vi "WaveFormDataGenerator.vi"(8 "error in":errorcluster, 9 "sampling info":cluster{"Fs":dbl, "#s":dbl}={"Fs"=1000.0, "#s"=100.0}, 10 "Signal Types/Classes":T1(array[ring])=[enum."Sine Wave", enum."Square Wave", enum."Triangle Wave"], 11 "Number of Waveforms per Signal Type":i32=2500) -> (0 "error out":errorcluster, 2 "One-Hot Encoded Labels":sgl[][](array[numeric]), 3 "Generated Waveform":sgl[][](array[numeric]))   [LabVIEW 2020]
uses:
  <vilib>/numeric/Random Number (Range) DBL.vi
  <vilib>/measure/NI_MABase.lvlib
  <vilib>/Ngene/DeepLTK/Toolkit/Deep_Learning_Toolkit_by_Ngene.lvlib
panel:
  out "Class Indices":i32[](array[numeric])
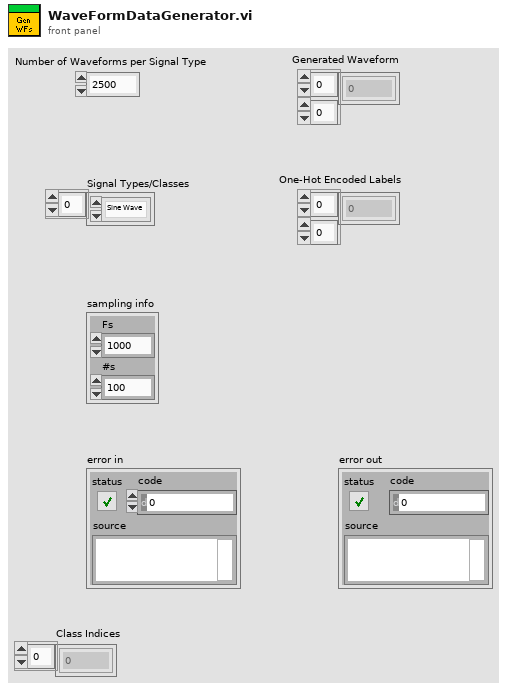
[diagram p1: front panel]
types:
  T1 = enum16{"Sine Wave", "Triangle Wave", "Square Wave", "Sawtooth Wave", "Noise"}[]
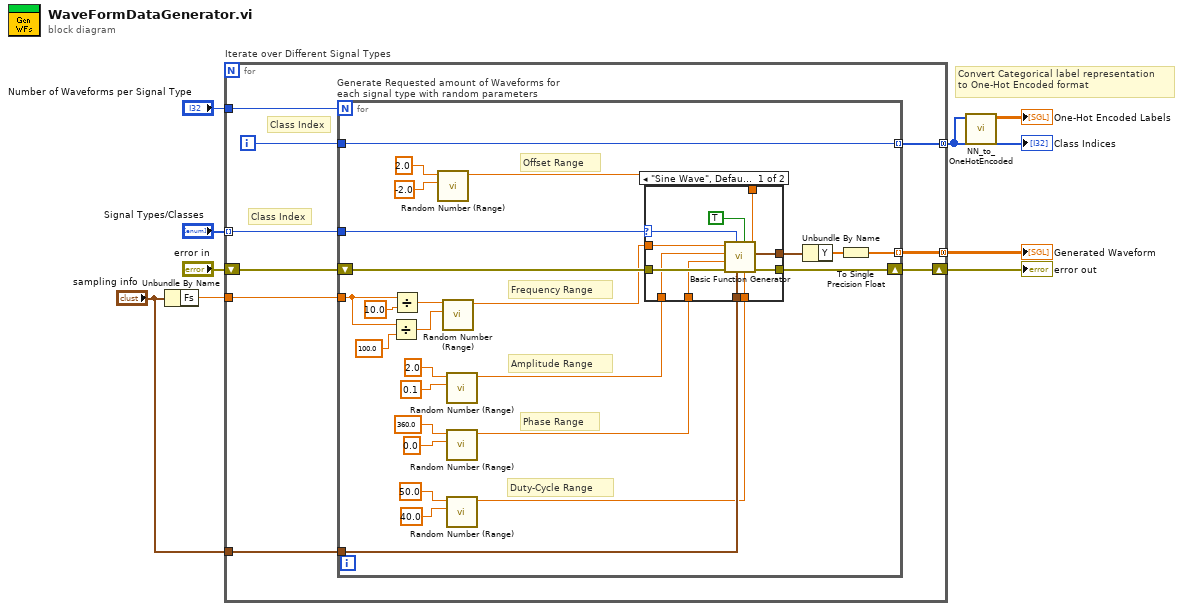
[diagram p0: block diagram]
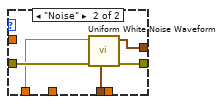
[diagram p2: hidden frame]
diagram:
  # "Convert Categorical label representation \nto One-Hot Encoded format"
  n1 = Unbundle By Name("sampling info") -> ("Fs"=w9:dbl)
  n2 = for "Iterate over Different Signal Types" {
    tunnel: w9 -> [w18]
    tunnel: "Number of Waveforms per Signal Type" -> [w17]
    tunnel: "sampling info" -> [w16]
    tunnel: [w13] -> w4 mode=concatenating
    tunnel: "Signal Types/Classes" -> [w12] mode=indexing
    shift-right: [w15] -> w6
    shift-left: "error in" -> [w14]
    tunnel: [w10] -> w2 mode=concatenating
    i -> [w11]
    # "Class Index"
    # "Class Index"
    n3 = for "Generate Requested amount of Waveforms for each signal type with random parameters" {
      N: w17 -> [_]
      tunnel: [w38] -> w13 mode=indexing
      shift-right: [w43] -> w15
      shift-left: w14 -> [w44]
      tunnel: w18 -> [w34]
      tunnel: w12 -> [w37]
      tunnel: w16 -> [w41]
      tunnel: [w36] -> w10 mode=indexing
      tunnel: w11 -> [w36]
      # "Offset Range"
      # "Duty-Cycle Range"
      # "Phase Range"
      # "Amplitude Range"
      # "Frequency Range"
      n4 = Divide(x=w34, y=100.0) -> (x/y=w33:dbl)
      n5 = Divide(x=w34, y=10.0) -> (x/y=w35:dbl)
      n6 = call-poly <vilib>:"Random Number (Range).vi"("lower bound (0)"=-2.0, "upper bound (100)"=2.0) -> ("number"=w19:dbl)  [unwired: 9 in]
      n7 = call-poly <vilib>:"Random Number (Range).vi"("lower bound (0)"=w33, "upper bound (100)"=w35) -> ("number"=w31:dbl)  [unwired: 9 in]
      n8 = call-poly <vilib>:"Random Number (Range).vi"("lower bound (0)"=0.1, "upper bound (100)"=2.0) -> ("number"=w28:dbl)  [unwired: 9 in]
      n9 = call-poly <vilib>:"Random Number (Range).vi"("lower bound (0)"=0.0, "upper bound (100)"=360.0) -> ("number"=w25:dbl)  [unwired: 9 in]
      n10 = call-poly <vilib>:"Random Number (Range).vi"("lower bound (0)"=40.0, "upper bound (100)"=50.0) -> ("number"=w22:dbl)  [unwired: 9 in]
      n11 = case shown="\"Sine Wave\", Default" w37 {
        selector: w37 -> [w50 _]
        tunnel: w44 -> [w55 w59]
        tunnel: [w54 w58] -> w43
        tunnel: w31 -> [w53 _]
        tunnel: w41 -> [w52 w60]
        tunnel: [w51 w57] -> w40
        tunnel: w28 -> [w49 w56]
        tunnel: w25 -> [w48 _]
        tunnel: w22 -> [w47 _]
        tunnel: w19 -> [w46 _]
        frame "Sine Wave", Default {
          n12 = call <vilib>:"Basic Function Generator.vi"("offset"=w46, "square wave duty cycle (%)"=w47, "reset signal"=TRUE, "sampling info"=w52, "signal type"=w50, "error in (no error)"=w55, "phase"=w48, "amplitude"=w49, "frequency"=w53) -> ("error out"=w54:errorcluster, "signal out"=w51:waveform(dbl))  [unwired: 1 out]
        }
        frame "Noise" {
          n13 = call <vilib>:"Uniform White Noise Waveform.vi"("sampling info"=w60, "error in (no error)"=w59, "amplitude"=w56) -> ("error out"=w58:errorcluster, "signal out"=w57:waveform(dbl))  [unwired: 7 in]
        }
      }
      n14 = Unbundle By Name(w40) -> ("Y"=w39:dbl[])
      n15 = To Single Precision Float(number=w39) -> (single precision float=w38:sgl[])
    }
  }
  "Generated Waveform" <- w4
  "error out" <- w6
  "Class Indices" <- w2
  n16 = call <vilib>:"NN_to_OneHotEncoded.vi"("Label_Idx"=w2) -> ("Prediction"=→"One-Hot Encoded Labels":sgl[][])  [unwired: 10 in]
